vi "Channel Set DataType.vi"(8 "error in (no error)":errorcluster, 10 "DataType":T1, 11 "Item Ref in":T2 format="%.0x") -> (0 "error out":errorcluster, 3 "Item Ref out":T2 format="%.0x")   [LabVIEW 2020, in "Modbus Master System Explorer.lvlib"]
uses:
  Modbus Master System Explorer.lvlib
  <vilib>/NI VeriStand/Custom Device API/Custom Device Item Ref.ctl
  Shared/Controls/Data Model/DataType.ctl
  Shared/Constants.vi
  <vilib>/NI VeriStand/Custom Device API/Set Item Property (U16).vi
  <vilib>/NI VeriStand/Custom Device API/Custom Device API.lvlib
  Shared/Modbus Master Shared.lvlib
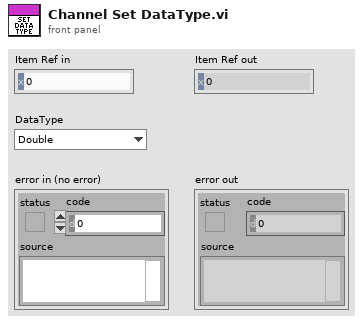
[diagram p1: front panel]
types:
  T1 = typedef "Modbus Master Shared.lvlib/DataType.ctl" = enum16{"Double", "Single", "I64", "I32", "I16", "I8", "U64", "U32", "U16", "U8", "Boolean"}
  T2 = typedef "Custom Device API.lvlib/Custom Device Item Ref.ctl" = u64
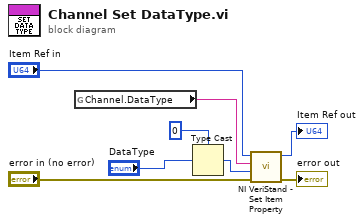
[diagram p0: block diagram]
diagram:
  n1 = global read "Constants.vi" "Channel.DataType"() -> (w8:string)
  n2 = Type Cast(type=u16 0, x="DataType") -> (*(type *) &x=w1:u16)
  n3 = call-poly <vilib>:"NI VeriStand - Set Item Property.vi"("error in (no error)"="error in (no error)", "Value"=w1, "Property Name"=w8, "Item Ref in"="Item Ref in") -> ("error out"=→"error out":errorcluster, "Item Ref out"=→"Item Ref out":T2)  [unwired: 5 in, 1 out]
